vi "Write Recipe.vi"(8 "error in (no error)":errorcluster, 10 "Recipe":refnum<class "Recipe.lvclass">, 11 "Cooker Actor in":refnum<class "Cooker Actor.lvclass">) -> (0 "error out":errorcluster, 3 "Cooker Actor out":refnum<class "Cooker Actor.lvclass">)   [LabVIEW 2024, in "Cooker Actor.lvlib" / "Cooker Actor.lvclass"]
uses:
  Cooker Actor.lvclass
  Cooker Actor.lvclass/Cooker Actor.ctl
  Support/Recipe/Recipe.lvclass
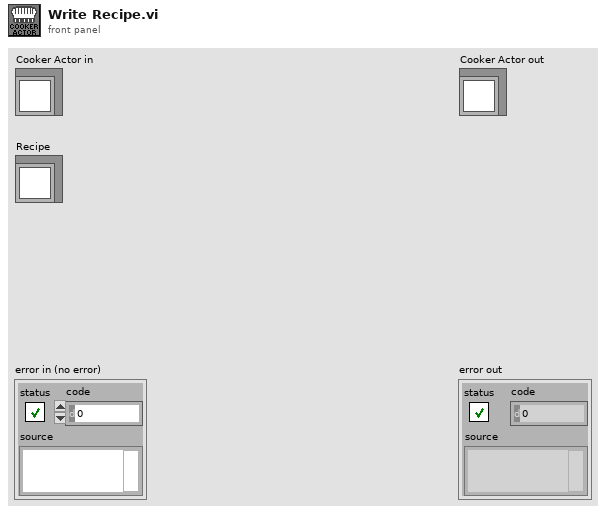
[diagram p1: front panel]
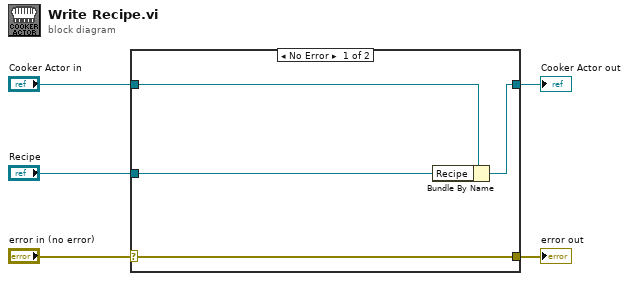
[diagram p0: block diagram]
diagram:
  n1 = case shown="No Error" "error in (no error)" {
    selector: "error in (no error)" -> [w9 w10]
    tunnel: [w9 w10] -> w4
    tunnel: [w7 w11] -> w2
    tunnel: "Cooker Actor in" -> [w8 w11]
    tunnel: "Recipe" -> [w6 _]
    frame No Error {
      n2 = Bundle By Name(cluster=w8, "Recipe"=w6) -> (w7:refnum<class "Cooker Actor.lvclass">)
    }
    frame Error {
    }
  }
  "error out" <- w4
  "Cooker Actor out" <- w2
